vi "read torque dvr.vi"(8 "error in (no error)":errorcluster, 11 "Torque Transducer in":refnum<class "Torque Transducer.lvclass">) -> (0 "error out":errorcluster, 1 "Torque":dbl, 2 "Time":timestamp, 3 "Torque Transducer out":refnum<class "Torque Transducer.lvclass">)   [LabVIEW 2025, in "Torque Transducer.lvclass"]
uses:
  Torque Transducer.lvclass
  Torque Transducer.lvclass/Torque Transducer.ctl
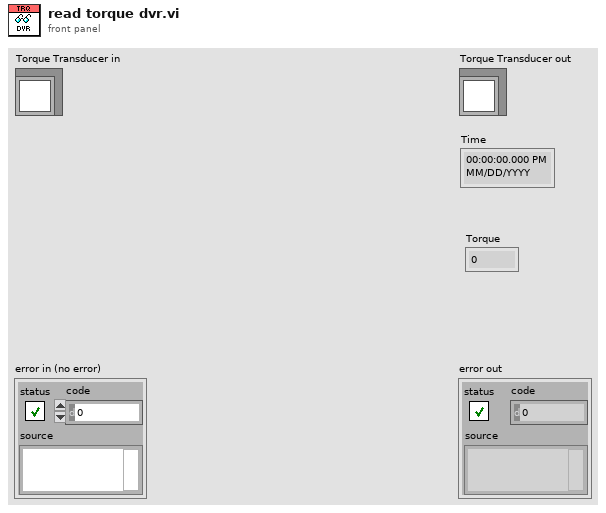
[diagram p1: front panel]
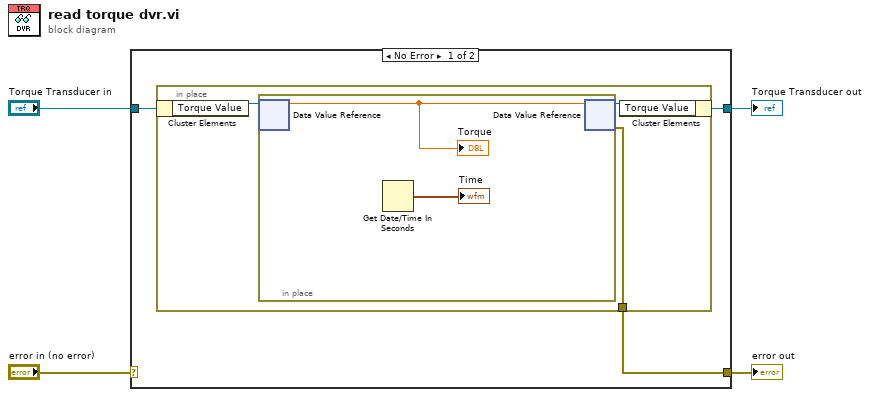
[diagram p0: block diagram]
diagram:
  n1 = case shown="No Error" "error in (no error)" {
    selector: "error in (no error)" -> [_ w14]
    tunnel: [w5 w14] -> w3
    tunnel: [w6 w13] -> w1
    tunnel: "Torque Transducer in" -> [w7 w13]
    frame No Error {
      n2 = in-place {
        in-place-border: [w8] -> w5
        n3 = in-place-cluster #1(w7) -> ("Torque Value"=w10:refnum<data-value>)
        n4 = in-place {
          n5 = in-place-dvr #2(w10) -> (w11:dbl)  [unwired: 1 out]
          "Torque" <- w11
          n6 = Get Date/Time In Seconds() -> (seconds since 1Jan1904=→"Time":timestamp)
          n7 = in-place-dvr #2(w11) -> (w9:refnum<data-value>, w8:errorcluster)
        }
        n8 = in-place-cluster #1("Torque Value"=w9) -> (w6:refnum<class "Torque Transducer.lvclass">)
      }
    }
    frame Error {
    }
  }
  "error out" <- w3
  "Torque Transducer out" <- w1
